vi "sqlite_generate_sql_insert_time.vi"(9 "Array":dbl[](array[numeric]), 10 "output cluster timestamp":timestamp, 11 "Array 2":string[](array[string])) -> (3 "String":string)   [LabVIEW 2011]
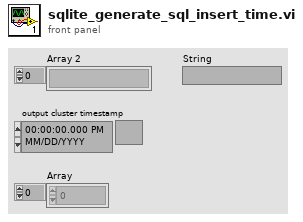
[diagram p1: front panel]
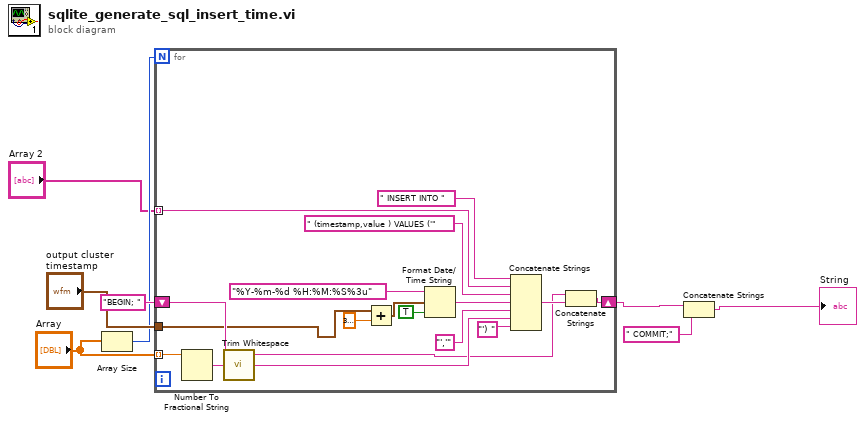
[diagram p0: block diagram]
diagram:
  n1 = Array Size(array="Array") -> (size(s)=w6:i32)
  n2 = for {
    N: w6 -> [_]
    tunnel: "Array" -> [w16] mode=indexing
    tunnel: "Array 2" -> [w15] mode=indexing
    shift-right: [w13] -> w3
    shift-left: "BEGIN; " -> [w12]
    tunnel: "output cluster timestamp" -> [w9]
    n3 = Number To Fractional String(number=w16) -> (F-format string=w23:string)  [unwired: 3 in]
    n4 = call <vilib>:"Trim Whitespace.vi"("string"=w23) -> ("trimmed string"=w24:string)  [unwired: 1 in]
    n5 = Add(x=w9, y=dbl[unit] 3600.0) -> (x+y=w11:timestamp)
    n6 = Format Date/Time String(time format string (%c)="%Y-%m-%d %H:%M:%S%3u", seconds (now)=w11, UTC format=TRUE) -> (date/time string=w21:string)
    n7 = Concatenate Strings(" INSERT INTO " ("SQL Query"), w15, " (timestamp,value ) VALUES ('" ("SQL Query"), w21, "','" ("string"), w24, "') " ("string")) -> (w14:string)
    n8 = Concatenate Strings(w12, w14) -> (w13:string)
  }
  n9 = Concatenate Strings(w3, " COMMIT;") -> (→"String":string)
